vi "dose_FMI.vi"(0 "Prime?":bool=TRUE, 1 "Final Ingredient?":bool=TRUE, 4 "RPMbaseline":i32=350, 5 "uL/stroke":dbl=5.0, 6 "RPM Derate":dbl=1.0, 7 "Volume (uL)":i32=1, 8 "OpenValve#":i32=1, 9 "RequestedValve#":i32) -> ()   [LabVIEW 2019]
panel:
  out "reverse":timestamp
  out "dose":timestamp
  out "prime":timestamp
  out "start":timestamp
  in  "NoPrimeFill":bool
  in  "Reverse Strokes":i32=27
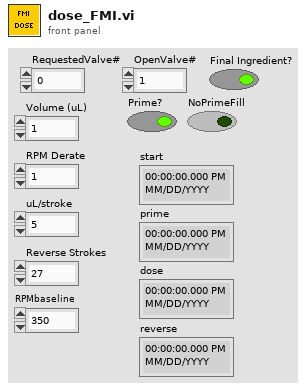
[diagram p1: front panel]
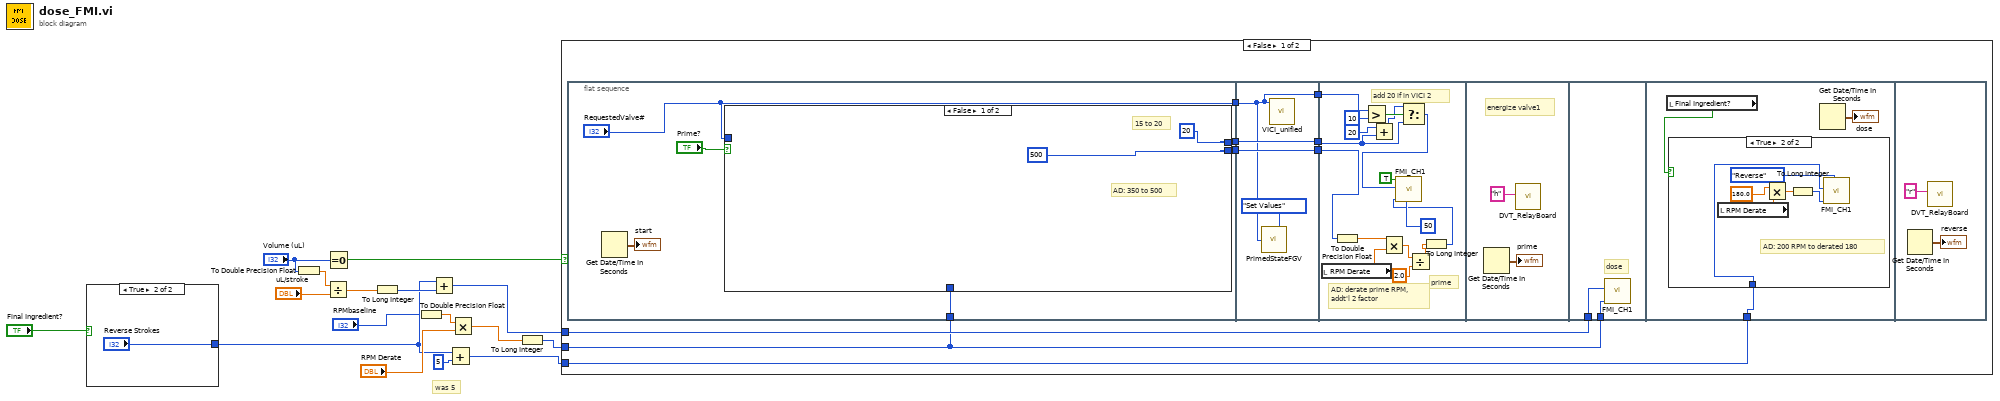
[diagram p0: block diagram]
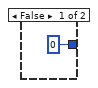
[diagram p2: hidden frame]
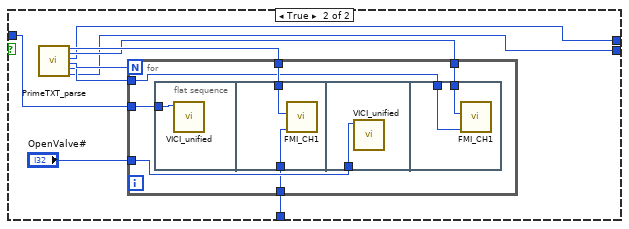
[diagram p3: hidden frame]
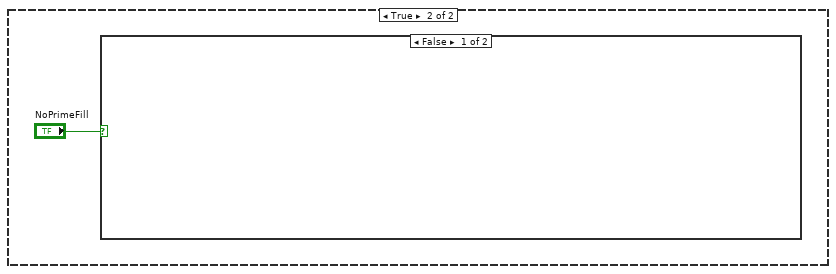
[diagram p5: hidden frame]
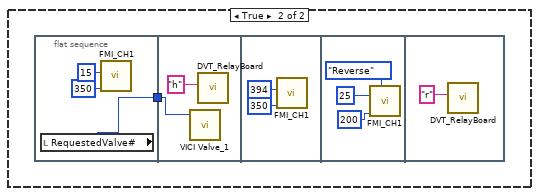
[diagram p6: hidden frame]
diagram:
  # "was 5"
  n1 = case shown="True" "Final Ingredient?" {
    tunnel: [0 ("Reverse Strokes") "Reverse Strokes"] -> w12
    frame False {
    }
    frame True {
    }
  }
  n2 = To Double Precision Float(number="Volume (uL)") -> (double precision float=w5:dbl)
  n3 = Divide(x=w5, y="uL/stroke") -> (x/y=w15:dbl)
  n4 = Equal To 0?(x="Volume (uL)") -> (x = 0?=w9:bool)
  n5 = To Long Integer(number=w15) -> (32bit integer=w14:i32)
  n6 = To Double Precision Float(number="RPMbaseline") -> (double precision float=w4:dbl)
  n7 = Add(x=w12, y=w14) -> (x+y=w13:i32)
  n8 = Add(x=w12, y=5) -> (x+y=w10:i32)
  n9 = Multiply(x=w4, y="RPM Derate") -> (x*y=w8:dbl)
  n10 = To Long Integer(number=w8) -> (32bit integer=w7:i32)
  n11 = case shown="False" w9 {
    tunnel: w7 -> [w22 _]
    tunnel: w13 -> [w24 _]
    tunnel: w10 -> [w23 _]
    frame False {
      n12 = flat-sequence {
        tunnel: ["RequestedValve#"] -> w27
        tunnel: [w31] -> w26
        tunnel: w22 -> [w30]
        tunnel: [w29] -> w20
        tunnel: w27 -> [w57]
        tunnel: [w60] -> w25
        tunnel: w26 -> [w60]
        tunnel: [w59] -> w21
        tunnel: w20 -> [w59]
        tunnel: [w57] -> w19
        tunnel: w25 -> [w71]
        tunnel: w21 -> [w65]
        tunnel: w19 -> [w73]
        tunnel: w22 -> [w80]
        tunnel: w24 -> [w79]
        tunnel: w23 -> [w83]
        frame #0 {
          n13 = Get Date/Time In Seconds() -> (seconds since 1Jan1904=→"start":timestamp)
          n14 = case shown="False" "Prime?" {
            tunnel: "RequestedValve#" -> [_ w44]
            tunnel: [20 ("Strokes") w39] -> w31
            tunnel: w30 -> [_ w42]
            tunnel: [500 ("RPM_prime") w36] -> w29
            frame False {
              # "15 to 20"
              # "AD: 350 to 500"
            }
            frame True {
              n15 = call "PrimeTXT_parse.vi"() -> ("Strokes_solvent"=w41:i32, "Strokes_air"=w40:i32, "Strokes_prime"=w39:i32, "Iterations"=w38:i32, "RPM_air"=w37:i32, "RPM_prime"=w36:i32)  [unwired: 13 in, 1 out]
              n16 = for {
                N: w38 -> [_]
                tunnel: w44 -> [w50]
                tunnel: "OpenValve#" -> [w49]
                tunnel: w42 -> [w48]
                tunnel: w41 -> [w47]
                tunnel: w40 -> [w46]
                tunnel: w37 -> [w45]
                n17 = flat-sequence {
                  tunnel: w50 -> [w51]
                  tunnel: w48 -> [w53]
                  tunnel: w47 -> [w52]
                  tunnel: w49 -> [w54]
                  tunnel: w46 -> [w56]
                  tunnel: w45 -> [w55]
                  frame #0 {
                    n18 = call "VICI_unified.vi"("RequestedValve#"=w51) -> ()  [unwired: 11 in]
                  }
                  frame #1 {
                    n19 = call "FMI_CH1.vi"("RPM"=w53, "Strokes"=w52) -> ()  [unwired: 6 in]
                  }
                  frame #2 {
                    n20 = call "VICI_unified.vi"("RequestedValve#"=w54) -> ()  [unwired: 11 in]
                  }
                  frame #3 {
                    n21 = call "FMI_CH1.vi"("RPM"=w55, "Strokes"=w56) -> ()  [unwired: 6 in]
                  }
                }
              }
            }
          }
        }
        frame #1 {
          n22 = call "PrimedStateFGV.vi"("Enum"=enum16{"Set Values", "Set Time", "Get Values"}."Set Values", "LastValve_write"=w57) -> ()  [unwired: 12 in, 2 out]
          n23 = call "VICI_unified.vi"("RequestedValve#"=w57) -> ()  [unwired: 11 in]
        }
        frame #2 {
          # "AD: derate prime RPM, addt'l 2 factor"
          # "add 20 if in VICI 2"
          # "prime"
          n24 = local read "RPM Derate"() -> (w67:dbl)
          n25 = To Double Precision Float(number=w65) -> (double precision float=w66:dbl)
          n26 = Greater?(x=w73, y=10) -> (0:w74:bool)
          n27 = Add(x=20, y=w71) -> (x+y=w69:i32)
          n28 = Multiply(x=w66, y=w67) -> (x*y=w63:dbl)
          n29 = Select(t=w69, s=w74, f=w71) -> (s? t:f=w68:i32)
          n30 = Divide(x=w63, y=2.0) -> (x/y=w61:dbl)
          n31 = To Long Integer(number=w61) -> (32bit integer=w64:i32)
          n32 = call "FMI_CH1.vi"("Accel"=50, "RPM"=w64, "Strokes"=w68, "Home Pump"=TRUE) -> ()  [unwired: 4 in]
        }
        frame #3 {
          # "energize valve1"
          n33 = Get Date/Time In Seconds() -> (seconds since 1Jan1904=→"prime":timestamp)
          n34 = call "DVT_RelayBoard.vi"("write buffer"="h") -> ()  [unwired: 3 in, 3 out]
        }
        frame #4 {
          # "dose"
          n35 = call "FMI_CH1.vi"("RPM"=w80, "Strokes"=w79) -> ()  [unwired: 6 in]
        }
        frame #5 {
          n36 = local read "Final Ingredient?"() -> (w81:bool)
          n37 = case shown="True" w81 {
            tunnel: w83 -> [_ w88]
            frame False {
            }
            frame True {
              # "AD: 200 RPM to derated 180"
              n38 = local read "RPM Derate"() -> (w85:dbl)
              n39 = Multiply(x=180.0 ("RPM"), y=w85) -> (x*y=w87:dbl)
              n40 = To Long Integer(number=w87) -> (32bit integer=w84:i32)
              n41 = call "FMI_CH1.vi"("Direction"=enum16{"Forward", "Reverse"}."Reverse", "RPM"=w84, "Strokes"=w88) -> ()  [unwired: 5 in]
            }
          }
          n42 = Get Date/Time In Seconds() -> (seconds since 1Jan1904=→"dose":timestamp)
        }
        frame #6 {
          n43 = Get Date/Time In Seconds() -> (seconds since 1Jan1904=→"reverse":timestamp)
          n44 = call "DVT_RelayBoard.vi"("write buffer"="r") -> ()  [unwired: 3 in, 3 out]
        }
      }
    }
    frame True {
      n45 = case shown="False" "NoPrimeFill" {
        frame False {
        }
        frame True {
          n46 = flat-sequence {
            tunnel: [w96] -> w93
            tunnel: w93 -> [w97]
            frame #0 {
              n47 = local read "RequestedValve#"() -> (w96:i32)
              n48 = call "FMI_CH1.vi"("RPM"=350, "Strokes"=15) -> ()  [unwired: 6 in]
            }
            frame #1 {
              n49 = call "VICI Valve_1.vi"("RequestedValve#"=w97) -> ()  [unwired: 2 in, 3 out]
              n50 = call "DVT_RelayBoard.vi"("write buffer"="h") -> ()  [unwired: 3 in, 3 out]
            }
            frame #2 {
              n51 = call "FMI_CH1.vi"("RPM"=350, "Strokes"=394) -> ()  [unwired: 6 in]
            }
            frame #3 {
              n52 = call "FMI_CH1.vi"("Direction"=enum16{"Forward", "Reverse"}."Reverse", "RPM"=200, "Strokes"=25) -> ()  [unwired: 5 in]
            }
            frame #4 {
              n53 = call "DVT_RelayBoard.vi"("write buffer"="r") -> ()  [unwired: 3 in, 3 out]
            }
          }
        }
      }
    }
  }
